vi "曲线状态.vi"(7 "枚举":enum16{"Read", "Write"}(ring), 11 "Status_Write":i16) -> (3 "Status_Read":i16)   [LabVIEW 2020]
uses:
  Libraries/S7/S7.lvlib
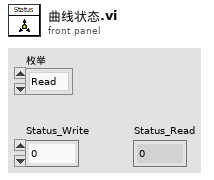
[diagram p1: front panel]
types:
  T1 = typedef "S7.lvlib/Read_Data (Reply Payload)--cluster.ctl" = cluster{"读取成功":bool, "数据":u32[], "Read_Data_error":errorcluster}
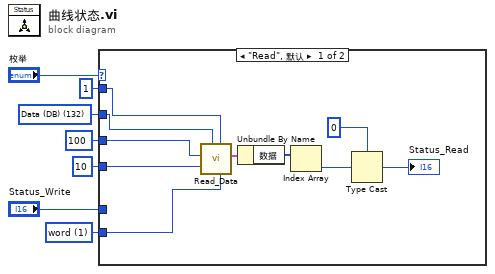
[diagram p0: block diagram]
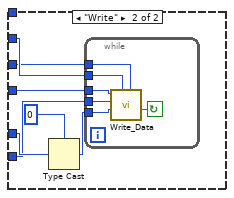
[diagram p2: hidden frame]
diagram:
  w3 = u16 1 items=["byte", "word", "Dword"] ("数据类型")
  w4 = u8 132 items=["I/O (P)"=128, "Input (I)"=129, "Output (Q)"=130, "Bit Memory (M)"=131, "Data (DB)"=132, "Instance Data (DI)"=133, "Local Data (L)"=134, "Predecessor Local Data (VL)"=135] ("寄存器类型")
  n1 = case shown="\"Read\", 默认" "枚举" {
    tunnel: u16 100 ("DB #") -> [w17 w19]
    tunnel: u32 10 ("起始地址") -> [w16 w18]
    tunnel: w4 -> [w15 w21]
    tunnel: u16 1 ("读取长度") -> [w14 _]
    tunnel: w3 -> [w13 w20]
    tunnel: "Status_Write" -> [_ w22]
    frame "Read", Default {
      n2 = call "Read_Data.vi"("数据类型"=w13, "读取长度"=w14, "寄存器类型"=w15, "起始地址"=w16, "DB #"=w17) -> ("Reply Payload"=w11:T1)  [unwired: 4 in, 2 out]
      n3 = Unbundle By Name(w11) -> ("数据"=w10:u32[])
      n4 = Index Array(array=w10) -> (element=w8:u32)  [unwired: 1 in]
      n5 = Type Cast(type=u32 0, x=w8) -> (*(type *) &x=→"Status_Read":u32)
    }
    frame "Write" {
      n6 = Type Cast(type=u16 0, x=w22) -> (*(type *) &x=w23:u16)
      n7 = while {
        tunnel: w23 -> [w30]
        tunnel: w21 -> [w29]
        tunnel: w20 -> [w28]
        tunnel: w19 -> [w27]
        tunnel: w18 -> [w26]
        stop <- w25 continue-if-true
        n8 = call "Write_Data.vi"("DB #"=w27, "寄存器类型"=w29, "写入数据"=w30, "数据类型"=w28, "写入地址"=w26) -> ("timed out?"=w25:bool)  [unwired: 4 in, 2 out]
      }
    }
  }
